vi "Remove Point.vi"(8 "error in (no error)":errorcluster, 11 "Outline in":refnum<class "Outline.lvclass">) -> (0 "error out":errorcluster, 3 "Outline out":refnum<class "Outline.lvclass">)   [LabVIEW 2013, in "Outline.lvclass"]
uses:
  Outline.lvclass
  Outline.lvclass/Outline.ctl
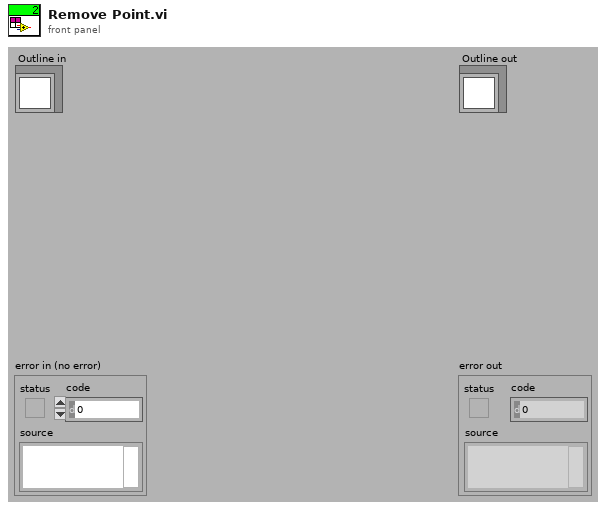
[diagram p1: front panel]
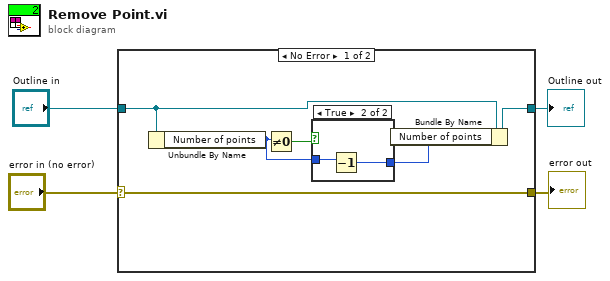
[diagram p0: block diagram]
diagram:
  n1 = case shown="No Error" "error in (no error)" {
    selector: "error in (no error)" -> [w10 w15]
    tunnel: [w10 w15] -> w3
    tunnel: [w5 w14] -> w1
    tunnel: "Outline in" -> [w6 w14]
    frame No Error {
      n2 = Unbundle By Name(w6) -> ("Number of points"=w8:i32)
      n3 = Not Equal To 0?(x=w8) -> (x != 0?=w9:bool)
      n4 = case shown="True" w9 {
        tunnel: w8 -> [w11 w13]
        tunnel: [w11 w12] -> w7
        frame False {
        }
        frame True {
          n5 = Decrement(x=w13) -> (x-1=w12:i32)
        }
      }
      n6 = Bundle By Name(cluster=w6, "Number of points"=w7) -> (w5:refnum<class "Outline.lvclass">)
    }
    frame Error {
    }
  }
  "error out" <- w3
  "Outline out" <- w1
